vi "Housekeeping.vi"(8 "error in":errorcluster, 10 "PAS Cell Data In":refnum<class "PAS Cell Data.lvclass">=refnum, 11 "PAS File Obs in":refnum<class "PAS File Obs.lvclass">) -> (0 "error out":errorcluster, 2 "PAS Cell Data Out":refnum<class "PAS Cell Data.lvclass">, 3 "PAS File Obs Out":refnum<class "PAS File Obs.lvclass">)   [LabVIEW 2014, in "PAS File Obs.lvclass"]
uses:
  PAS File Obs.lvclass
  Main/Controls/Cell Data.ctl
  Data/Cell/PAS Cell Data.lvclass
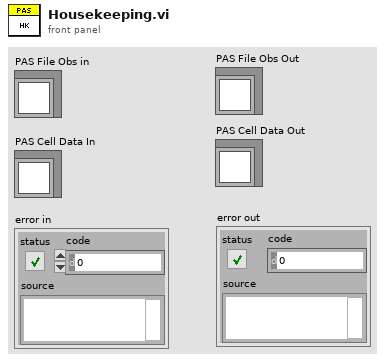
[diagram p1: front panel]
types:
  T1 = enum16{"big-endian, network order", "native, host order", "little-endian"}
  T2 = typedef "Cell Data.ctl" = u8
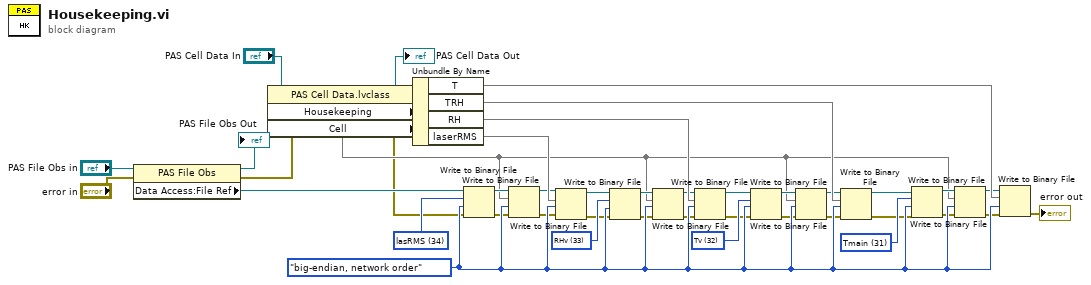
[diagram p0: block diagram]
diagram:
  w38 = T1."big-endian, network order" ("byte order (0:big-endian, network order)")
  w37 = T2 31 items=["TEC SP"=23, "TEC Enable"=24, "Qsp"=25, "Tac"=26, "Pac"=27, "Q0ac"=28, "Qac"=29, "Cell TEC T (T1)"=30, "Tmain"=31, "Tv"=32, "RHv"=33, "lasRMS"=34, "dPhi"=35, "Tau"=36, "Cell Q"=37, "f0"=38, "Integrated Area"=39, "Max Amplitude"=40, "Noise Limit"=41, "Lower Noise Bound"=42, "Upper Noise Bound"=43, "Absorption"=44, "fit params"=45, "covariance"=46] ("cellNumData")
  w30 = T2 32 items=["TEC SP"=23, "TEC Enable"=24, "Qsp"=25, "Tac"=26, "Pac"=27, "Q0ac"=28, "Qac"=29, "Cell TEC T (T1)"=30, "Tmain"=31, "Tv"=32, "RHv"=33, "lasRMS"=34, "dPhi"=35, "Tau"=36, "Cell Q"=37, "f0"=38, "Integrated Area"=39, "Max Amplitude"=40, "Noise Limit"=41, "Lower Noise Bound"=42, "Upper Noise Bound"=43, "Absorption"=44, "fit params"=45, "covariance"=46] ("cellNumData")
  w23 = T2 33 items=["TEC SP"=23, "TEC Enable"=24, "Qsp"=25, "Tac"=26, "Pac"=27, "Q0ac"=28, "Qac"=29, "Cell TEC T (T1)"=30, "Tmain"=31, "Tv"=32, "RHv"=33, "lasRMS"=34, "dPhi"=35, "Tau"=36, "Cell Q"=37, "f0"=38, "Integrated Area"=39, "Max Amplitude"=40, "Noise Limit"=41, "Lower Noise Bound"=42, "Upper Noise Bound"=43, "Absorption"=44, "fit params"=45, "covariance"=46] ("cellNumData")
  w16 = T2 34 items=["TEC SP"=23, "TEC Enable"=24, "Qsp"=25, "Tac"=26, "Pac"=27, "Q0ac"=28, "Qac"=29, "Cell TEC T (T1)"=30, "Tmain"=31, "Tv"=32, "RHv"=33, "lasRMS"=34, "dPhi"=35, "Tau"=36, "Cell Q"=37, "f0"=38, "Integrated Area"=39, "Max Amplitude"=40, "Noise Limit"=41, "Lower Noise Bound"=42, "Upper Noise Bound"=43, "Absorption"=44, "fit params"=45, "covariance"=46] ("cellNumData")
  n1 = property class="PAS File Obs"(reference="PAS File Obs in", error in="error in") -> (reference out=→"PAS File Obs Out":refnum<class "PAS File Obs.lvclass">, error out=w5:errorcluster, "Data Access:File Ref"=w10:refnum<file>)
  n2 = property class="PAS Cell Data.lvclass"(reference="PAS Cell Data In", error in=w5) -> (reference out=→"PAS Cell Data Out":refnum<class "PAS Cell Data.lvclass">, error out=w4:errorcluster, "Housekeeping"=w8, "Cell"=w7)
  n3 = Unbundle By Name(w8) -> ("T"=w39, "TRH"=w40, "RH"=w41, "laserRMS"=w42)
  n4 = Write to Binary File(file (use dialog)=w10, data=w16, error in=w4, 9:w38) -> (refnum out=w12:refnum<file>, error out=w13:errorcluster)  [unwired: 2 in, 1 out]
  n5 = Write to Binary File(file (use dialog)=w12, data=w7, error in=w13, 9:w38) -> (refnum out=w14:refnum<file>, error out=w15:errorcluster)  [unwired: 2 in, 1 out]
  n6 = Write to Binary File(file (use dialog)=w14, data=w42, error in=w15, 9:w38) -> (refnum out=w17:refnum<file>, error out=w18:errorcluster)  [unwired: 2 in, 1 out]
  n7 = Write to Binary File(file (use dialog)=w17, data=w23, error in=w18, 9:w38) -> (refnum out=w19:refnum<file>, error out=w20:errorcluster)  [unwired: 2 in, 1 out]
  n8 = Write to Binary File(file (use dialog)=w19, data=w7, error in=w20, 9:w38) -> (refnum out=w21:refnum<file>, error out=w22:errorcluster)  [unwired: 2 in, 1 out]
  n9 = Write to Binary File(file (use dialog)=w21, data=w41, error in=w22, 9:w38) -> (refnum out=w25:refnum<file>, error out=w24:errorcluster)  [unwired: 2 in, 1 out]
  n10 = Write to Binary File(file (use dialog)=w25, data=w30, error in=w24, 9:w38) -> (refnum out=w27:refnum<file>, error out=w26:errorcluster)  [unwired: 2 in, 1 out]
  n11 = Write to Binary File(file (use dialog)=w27, data=w7, error in=w26, 9:w38) -> (refnum out=w29:refnum<file>, error out=w28:errorcluster)  [unwired: 2 in, 1 out]
  n12 = Write to Binary File(file (use dialog)=w29, data=w40, error in=w28, 9:w38) -> (refnum out=w32:refnum<file>, error out=w31:errorcluster)  [unwired: 2 in, 1 out]
  n13 = Write to Binary File(file (use dialog)=w32, data=w37, error in=w31, 9:w38) -> (refnum out=w33:refnum<file>, error out=w34:errorcluster)  [unwired: 2 in, 1 out]
  n14 = Write to Binary File(file (use dialog)=w33, data=w7, error in=w34, 9:w38) -> (refnum out=w35:refnum<file>, error out=w36:errorcluster)  [unwired: 2 in, 1 out]
  n15 = Write to Binary File(file (use dialog)=w35, data=w39, error in=w36, 9:w38) -> (error out=→"error out":errorcluster)  [unwired: 2 in, 2 out]
